vi "Open FPGA.vi"(8 "error in (no error)":errorcluster, 9 "Channel Number":u32, 10 "Bitfile path":path=path "c:/ni-rt/VeriStand/Custom Devices/FPGA Addon/985xsupport_FPGATarget_fpga-main_5XgmTEdlmQU.lvbitx", 11 "Device address":string="RIO0") -> (0 "error out":errorcluster, 3 "Bitfile reference out":T1)   [LabVIEW 2020, in "985x Support Addon Engine.lvlib"]
uses:
  985x Support Addon Engine.lvlib
  Types/FPGA Refnum.ctl
  <vilib>/Utility/error.llb/Error Cluster From Error Code.vi
  <vilib>/ErrorRing/Error Ring.xnode
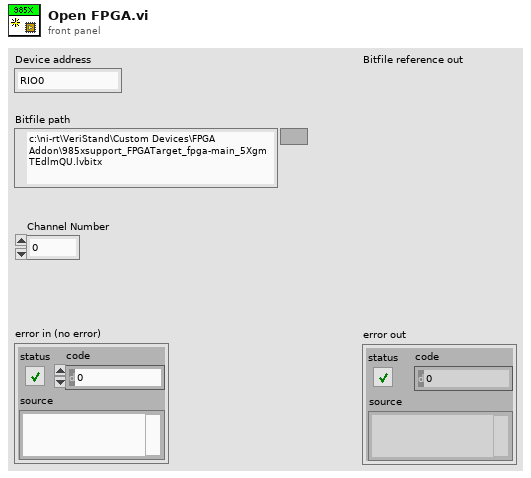
[diagram p1: front panel]
types:
  T1 = typedef "985x Support Addon Engine.lvlib/FPGA Refnum.ctl" = refnum<k20>
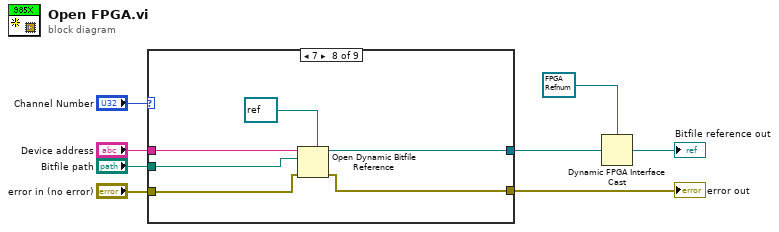
[diagram p0: block diagram]
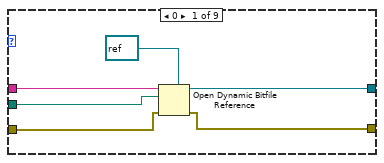
[diagram p2: hidden frame]
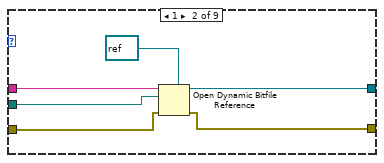
[diagram p3: hidden frame]
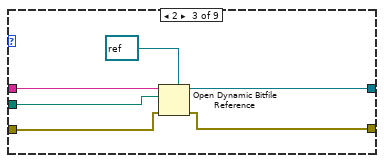
[diagram p4: hidden frame]
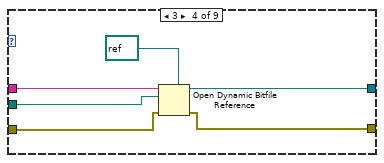
[diagram p5: hidden frame]
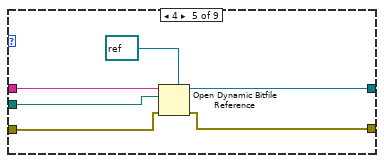
[diagram p6: hidden frame]
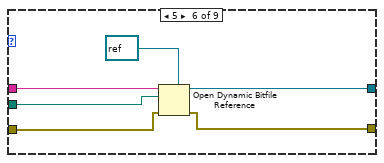
[diagram p7: hidden frame]
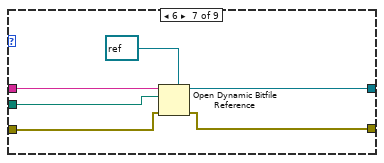
[diagram p8: hidden frame]
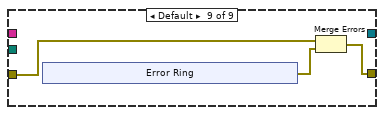
[diagram p9: hidden frame]
diagram:
  n1 = case shown="7" "Channel Number" {
    tunnel: [w14 w20 w26 w32 w38 w44 w50 w56 _] -> w7
    tunnel: "Device address" -> [w13 w19 w25 w31 w37 w43 w49 w55 _]
    tunnel: "Bitfile path" -> [w12 w18 w24 w30 w36 w42 w48 w54 _]
    tunnel: "error in (no error)" -> [w11 w17 w23 w29 w35 w41 w47 w53 w59]
    tunnel: [w10 w16 w22 w28 w34 w40 w46 w52 w57] -> w2
    frame 0 {
      n2 = Open Dynamic Bitfile Reference(0:w13, 1:w12, 3:w11, 4:refnum<k20> refnum ("Template")) -> (5:w14:refnum<k20>, 8:w10:errorcluster)  [unwired: 1 in]
    }
    frame 1 {
      n3 = Open Dynamic Bitfile Reference(0:w19, 1:w18, 3:w17, 4:refnum<k20> refnum ("Template")) -> (5:w20:refnum<k20>, 8:w16:errorcluster)  [unwired: 1 in]
    }
    frame 2 {
      n4 = Open Dynamic Bitfile Reference(0:w25, 1:w24, 3:w23, 4:refnum<k20> refnum ("Template")) -> (5:w26:refnum<k20>, 8:w22:errorcluster)  [unwired: 1 in]
    }
    frame 3 {
      n5 = Open Dynamic Bitfile Reference(0:w31, 1:w30, 3:w29, 4:refnum<k20> refnum ("Template")) -> (5:w32:refnum<k20>, 8:w28:errorcluster)  [unwired: 1 in]
    }
    frame 4 {
      n6 = Open Dynamic Bitfile Reference(0:w37, 1:w36, 3:w35, 4:refnum<k20> refnum ("Template")) -> (5:w38:refnum<k20>, 8:w34:errorcluster)  [unwired: 1 in]
    }
    frame 5 {
      n7 = Open Dynamic Bitfile Reference(0:w43, 1:w42, 3:w41, 4:refnum<k20> refnum ("Template")) -> (5:w44:refnum<k20>, 8:w40:errorcluster)  [unwired: 1 in]
    }
    frame 6 {
      n8 = Open Dynamic Bitfile Reference(0:w49, 1:w48, 3:w47, 4:refnum<k20> refnum ("Template")) -> (5:w50:refnum<k20>, 8:w46:errorcluster)  [unwired: 1 in]
    }
    frame 7 {
      n9 = Open Dynamic Bitfile Reference(0:w55, 1:w54, 3:w53, 4:refnum<k20> refnum ("Template")) -> (5:w56:refnum<k20>, 8:w52:errorcluster)  [unwired: 1 in]
    }
    frame Default {
      n10 = xnode "Error Ring"() -> ("error out"=w58:errorcluster)
      n11 = Merge Errors(w59, w58) -> (w57:errorcluster)
    }
  }
  "error out" <- w2
  n12 = Dynamic FPGA Interface Cast(Session In=T1 refnum ("FPGA Refnum"), Type=w7) -> (Session Out=→"Bitfile reference out":T1)
